vi "Dashboard Main.vi"() -> ()   [LabVIEW 2017]
uses:
  <vilib>/Utility/miscctls.llb/LVRowAndColumnTypeDef.ctl
  <vilib>/event_ctls.llb/eventvkey.ctl
  <vilib>/Rock Robotics/Network Tables/NT Read Numeric Array.vi
  <vilib>/Rock Robotics/WPI/Dashboard/WPI_DashboardLogging Global.vi
panel:
  in  "Camera Settings Right":T1={"Frame Rate"=30, "Compression"=30, "Size"=1, "DB Camera Config"=FALSE} {"Frame Rate" scale=1.0..30.0; "Compression" scale=100.0..-1.0; "Size" items=["640x480", "320x240", "160x120"]}
  in  "Camera Name Right":string(combo)="No Camera Selection"
  out "Camera Info":cluster{"Mbps LED":bool, "Mbps":dbl, "fps":dbl} {"fps" format="%#.1g"; "Mbps" format="%#.1g"}
  in  "Camera Settings":T1={"Frame Rate"=30, "Compression"=30, "Size"=1, "DB Camera Config"=FALSE} {"Frame Rate" scale=1.0..30.0; "Compression" scale=100.0..-1.0; "Size" items=["640x480", "320x240", "160x120"]}
  in  "TCP":refnum<k5>
  in  "Rec Mode":enum32{"Stop", "Record", "Playback"}(radio)
  out "Robot IP":string
  out "Image Message":string="Timeout in Camera Communications"
  in  "Dashboard Tab":T2(tab)
  out "Pitch":dbl
  out "Roll":dbl
  in  "Select Auto":string(combo)="Select Autonomous ..."
  out "NT Connection":bool
  out "MotorChart R":cluster{"Numeric":dbl, "Numeric":dbl}(graph)
  out "MotorChart L":cluster{"Numeric":dbl, "Numeric":dbl}(graph)
  out "MotorSliders R":cluster{"MotorSlide1":dbl, "MotorSlide2":dbl} {"MotorSlide2" scale=-1.0..1.0 scale format="%#_2e"; "MotorSlide1" scale=-1.0..1.0 scale format="%#_2e"}
  out "MotorSliders L":cluster{"MotorSlide1":dbl, "MotorSlide2":dbl} {"MotorSlide2" scale=-1.0..1.0 scale format="%#_2e"; "MotorSlide1" scale=-1.0..1.0 scale format="%#_2e"}
  out "Yaw":dbl
  out "JS1 Z":dbl(slide) scale=-1.0..1.0 scale format="%#_2e"
  out "JS1 Graph":cluster{"X":dbl, "Y":dbl}[](graph)
  out "JS1 Buttons":T3
  out "JS2 Z":dbl(slide) scale=-1.0..1.0 scale format="%#_2e"
  out "JS2 Graph":cluster{"X":dbl, "Y":dbl}[](graph)
  out "JS2 Buttons":T3
  out "Mode":T4(ring)=enum."Auto Disabled"
  out "Camera Image Right":T5(plugin-control)
  in  "DB/String 9":string
  in  "DB/String 8":string
  in  "DB/String 7":string
  in  "DB/String 6":string
  in  "DB/String 5":string
  in  "DB/String 4":string
  in  "DB/String 3":string
  in  "DB/String 2":string
  in  "DB/String 1":string
  in  "DB/String 0":string
  in  "DB/Slider 0":dbl(slide) scale=0.0..5.0
  in  "DB/Slider 1":dbl(slide) scale=0.0..5.0
  in  "DB/Slider 2":dbl(slide) scale=0.0..5.0
  in  "DB/Slider 3":dbl(slide) scale=0.0..5.0
  out "DB/LED 3":bool
  out "DB/LED 2":bool
  out "DB/LED 1":bool
  out "DB/LED 0":bool
  in  "DB/Button 3":bool
  in  "DB/Button 2":bool
  in  "DB/Button 1":bool
  in  "DB/Button 0":bool caption="New Name"
  in  "Test Slider":dbl(slide) scale=0.0..100.0 scale format="%#_3g"
  in  "On/Off":bool caption="Solenoid"
  in  "Test Name":u16(ring) items=["Select the test to run..."]
  in  "Test Tree":string(tree)
  in  "Motor":cluster{"Value":dbl, "Enable":bool} {"Value" scale=-1.0..1.0 scale format="%#_3g"}
  out "Progress":T6 {"Test Progress" scale=0.0..100.0}
  in  "Rev/Fwd":cluster{"Forward":bool, "Reverse":bool}
  in  "Test Ring":u16(ring) items=["Monochrome", "Color"]
  out "Cmd Status":string
  in  "Execute Command":bool
  in  "Command Params":string[][](table)
  in  "Command Selection":i32(listbox)
  in  "CheckList":i32(listbox)
  out "Tree":string(tree)
  out "Camera Image":T5(plugin-control)
  out "Background":bool
  in  "Camera Name":string(combo)="No Camera Selection"
  # "HW"
  # "HW"
  # "Joysticks"
  # "Drive Motors"
  # "Front"
  # "Right"
  # "Left"
  # "Back"
  # "This tab is a great place for autonomous settings and robot-specific values.\nPlace controls and indicators inside this tab and match name to\nDashboard Variables on robot. You can also delete this comment."
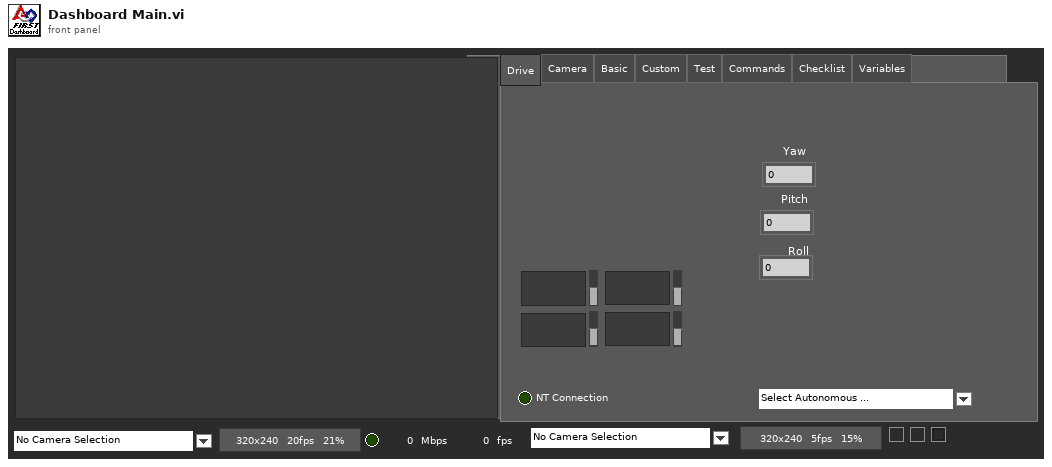
[diagram p1: front panel]
types:
  T1 = cluster{"Frame Rate":i32, "Compression":i32, "Size":u16, "DB Camera Config":bool}
  T2 = enum32{"Drive", "Camera", "Basic", "Custom", "Test", "Commands", "Checklist", "Variables"}
  T3 = cluster{bool, bool, bool, bool, bool, bool, bool, bool, bool, bool, bool, bool}
  T4 = enum8{"Tele-Op Disabled", "Tele-Op Enabled", "Auto Disabled", "Auto Enabled", "Test Disabled", "Test Enabled", "Disconnected", "No Code", "E-Stop"}
  T5 = typedef "IMAQ Image.ctl" = refnum<image>
  T6 = cluster{"Test Progress":u8, "Test Progress Text":string}
  T7 = cluster{"Save Path":path, "Interval (s)":dbl, "Keep":i32}
  T8 = typedef "Image Type" = u32
  T9 = cluster{"IDs":cluster{"RPC field ID":u16, "Unique ID":u16}, "String":string}
  T10 = cluster{"Camera Name":string, string, "Saved DB Images Info":cluster{"Save Path":path, "Interval (s)":dbl, "Keep":i32}}
  T11 = cluster{"Camera Name Right":string, string, "Saved DB Images Info":cluster{"Save Path":path, "Interval (s)":dbl, "Keep":i32}}
  T12 = cluster{"Camera Image":refnum<vi>, "Dashboard Tab":refnum<vi>, "Background":refnum<vi>, "Rec Mode":refnum<vi>, "Test Slider":refnum<vi>, "On/Off ":refnum<vi>, "Test Ring":refnum<vi>, "Rev/Fwd":refnum<vi>, "Test Name":refnum<vi>, "Motor":refnum<vi>, "Progress":refnum<vi>, "CheckList":refnum<vi>, "Tree":refnum<vi>, "Test Tree":refnum<vi>, "Command Params":refnum<vi>, "Command Selection":refnum<vi>, "Execute Command":refnum<vi>, "Cmd Status":refnum<vi>, "Camera Settings":refnum<vi>, "Camera Name":refnum<vi>, "Camera Info":refnum<vi>, "Camera Settings Right":refnum<vi>, "Camera Name Right":refnum<vi>, "Camera Image Right":refnum<vi>}
  T13 = cluster{"Error Strings":string, "Disable Counts":cluster{u16, u16}, "Rail Faults":cluster{u16, u16, u16}, "Robot IP":string, "DB Mode":u8, "Event Info":cluster{"Name":string, "Type":u8, "Number":u16, "Replay":u8}}
  T14 = cluster{"Storage":cluster{"Disk Free":u64, "RAM Block":u32, "RAM free":u32}, "CPU Utilization":cluster{"CPU % ISR":sgl, "CPU % Time Crit":sgl, "CPU % Timed Str":sgl, "CPU % High":sgl, "CPU % Above":sgl, "CPU % Normal":sgl, "CPU % Low":sgl}, "CAN":cluster{"% Bus Utilization":sgl, "Bus Off Cnt":u32, "TX_FIFO Full Cnt":u32, "Receive Error Cnt":u8, "Transmit Error Cnt":u8}, "HID":cluster{"HID Outputs":u32, "Rumble Low":u16, "Rumble High":u16}[]}
  T15 = cluster{"Status bits":cluster{"Test Mode":bool, "Autonomous":bool, "Enabled":bool, "Code Start":bool, "Brownout":bool, "Reserved 2":bool, "Reserved 3":bool, "E-Stop":bool}, "Code Trace":cluster{"Disabled":bool, "TeleOp":bool, "Auto":bool, "Test":bool}, "Controller Type":enum16{"unknown", "cRIO", "roboRio"}, "Code?":enum16{"unknown", "noCode", "code"}, "Battery V":dbl}
  T16 = cluster{"Control Bits":cluster{"TestMode":bool, "Autonomous":bool, "Enabled":bool, "FMS Present":bool, bool, bool, bool, "E-Stop":bool}, "Team Station ":u8, "Countdown":sgl, "Joystick Values":cluster{"Axes":dbl[], "Buttons":bool[], "POVs":i16[]}[]}
  T17 = cluster{"Axes":dbl[], "Buttons":bool[], "POVs":i16[]}[]
  T18 = cluster{"Axes":dbl[], "Buttons":bool[], "POVs":i16[]}
  T19 = cluster{"Buttons[0]":bool, "Buttons[1]":bool, "Buttons[2]":bool, "Buttons[3]":bool, "Buttons[4]":bool, "Buttons[5]":bool, "Buttons[6]":bool, "Buttons[7]":bool, "Buttons[8]":bool, "Buttons[9]":bool, "Buttons[10]":bool, "Buttons[11]":bool}
  T20 = cluster{"Operation":enum16{"Update", "Clear"}, "Color Box":u32}[]
  T21 = typedef "eventvkey.ctl" = enum16{"ASCII", "Enter", "Return", "Shift", "Ctrl", "Alt", "Cmd", "Opt", "Caps", "NumLock", "Clear", "Break", "Up", "Down", "Left", "Right", "Insert", "Delete", "Home", "End", "PageUp", "PageDown", "Escape", "Help", "Pause", "ScrollLock", "F1", "F2", "F3", "F4", "F5", "F6", "F7", "F8", "F9", "F10", "F11", "F12", "F13", "F14", "F15", "F16", "F17", "F18", "F19", "F20", "F21", "F22", "F23", "F24", "Play", "VolumeUp", "VolumeDown", "Mute", "Two Byte Char"}
  T22 = cluster{"Image Size":bool, "Image Type":bool, "Pixel Value":bool, "ROI Information":bool, "Zoom Factor":bool}
  T23 = cluster{"Operation":enum16{"Update", "Clear"}, "Color Box":u32}
  T24 = typedef "LVRowAndColumnTypeDef.ctl" = cluster{"Row":i32, "Column":i32}
  T25 = cluster{"Shift":bool, "Ctrl":bool, "Alt":bool, "Cmd":bool, "Opt":bool}
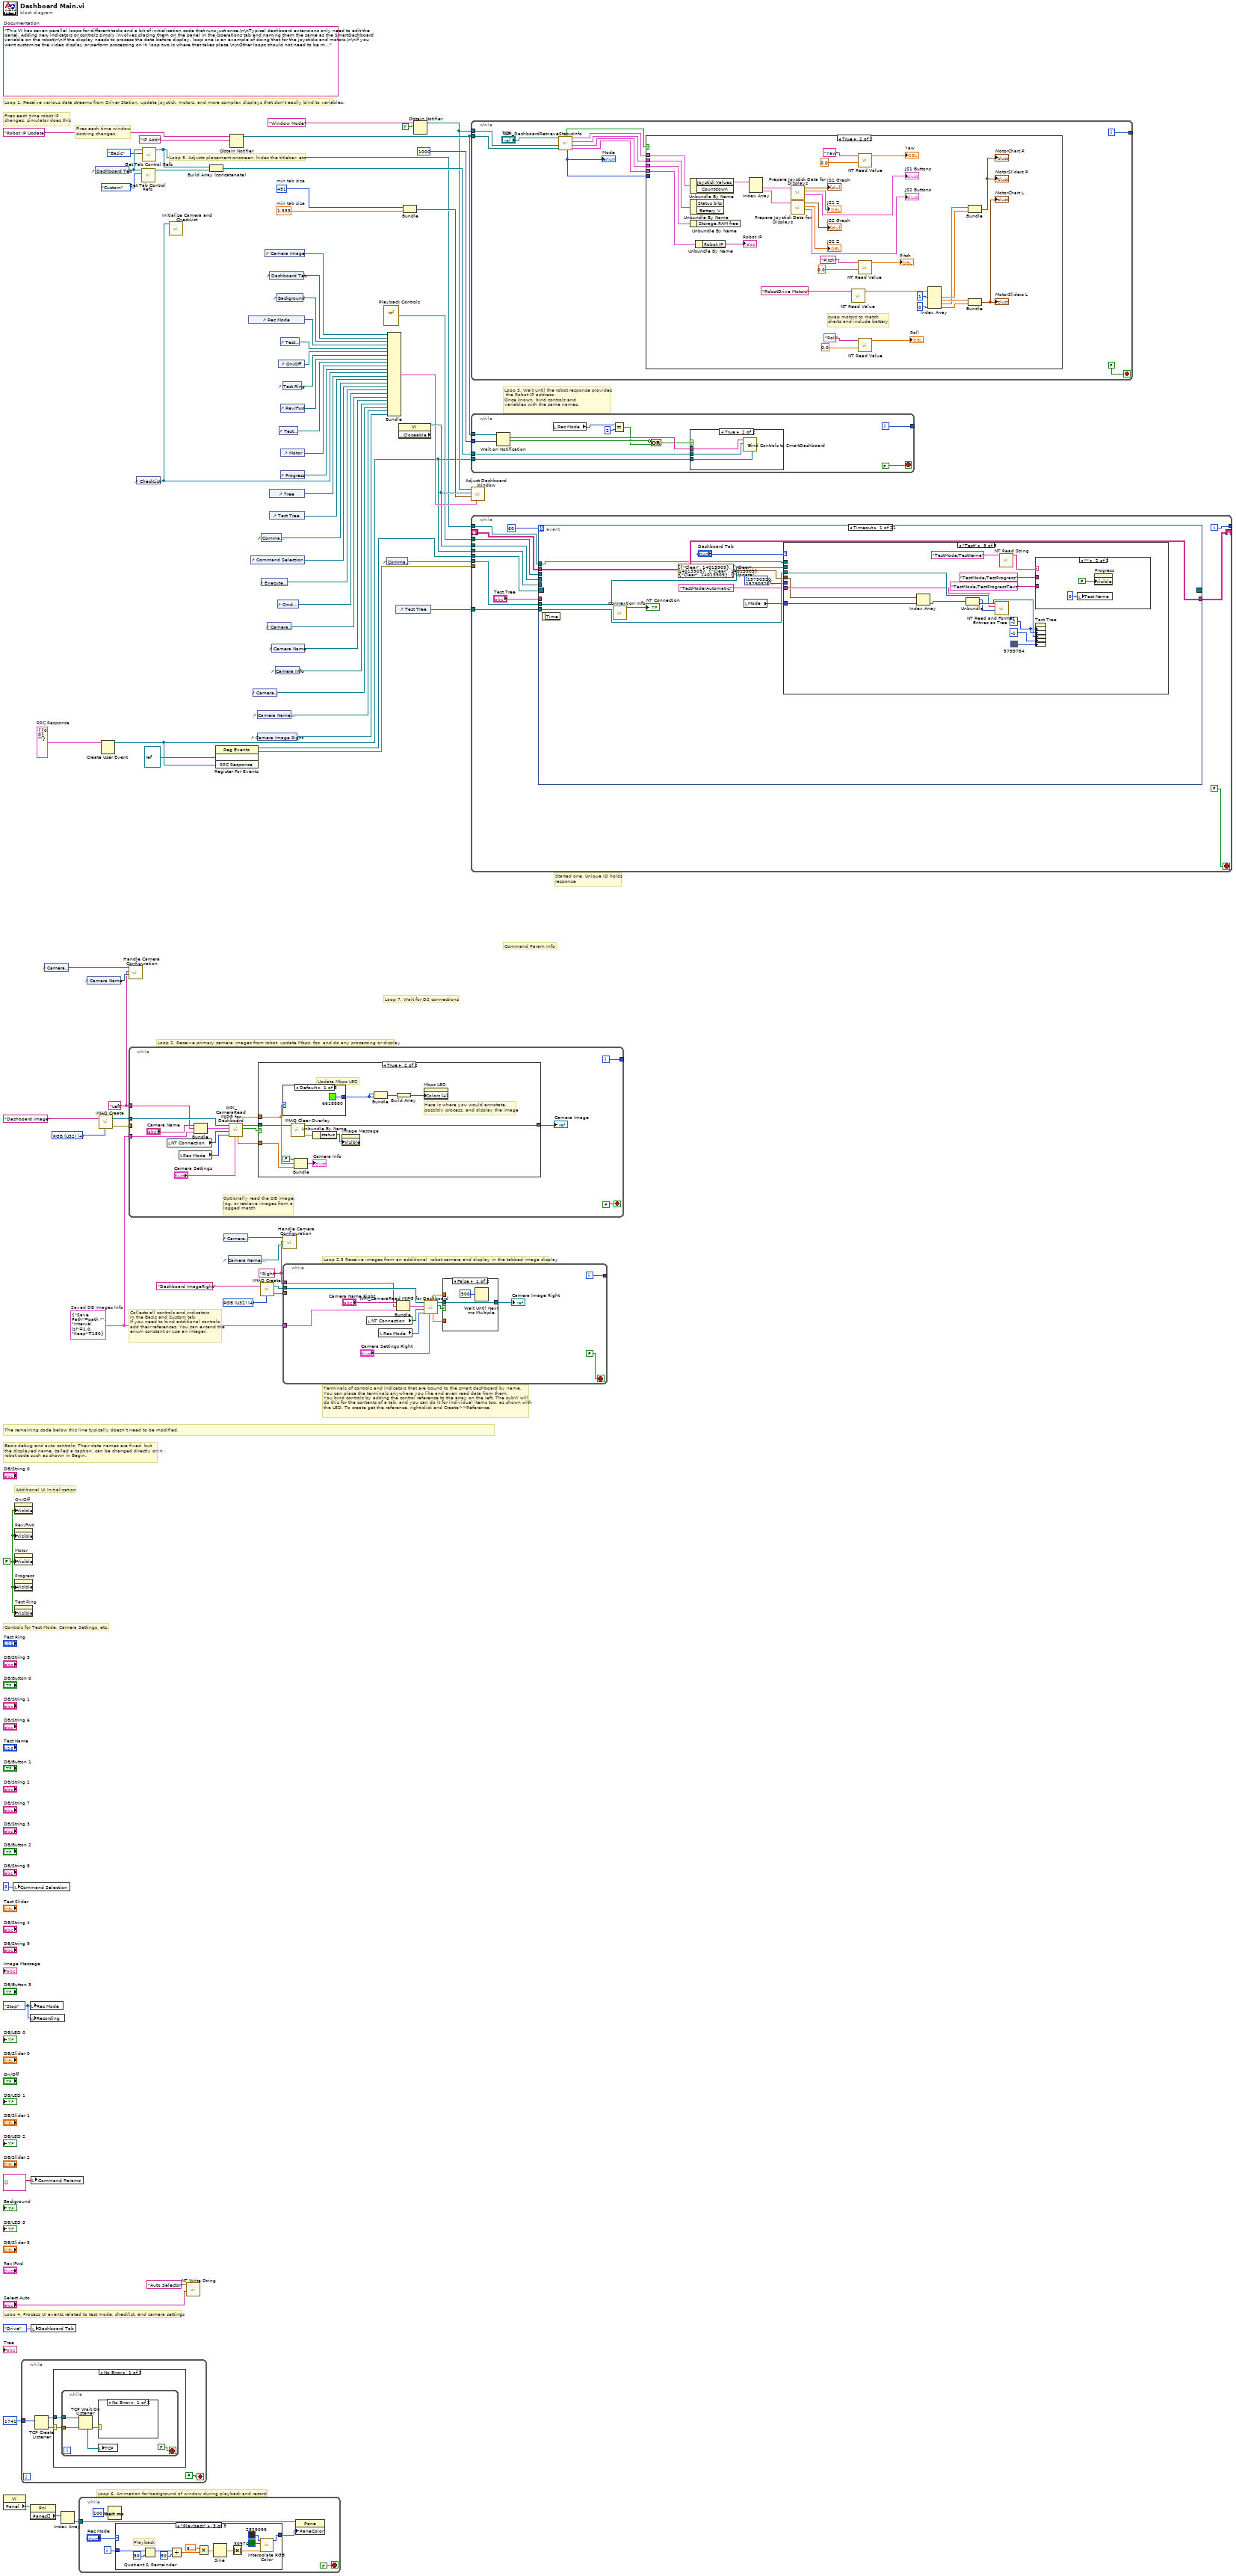
[diagram p0: block diagram]
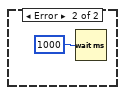
[diagram p3: hidden frame]
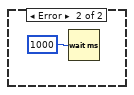
[diagram p4: hidden frame]
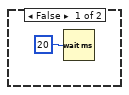
[diagram p5: hidden frame]
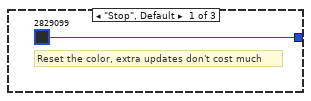
[diagram p6: hidden frame]
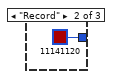
[diagram p7: hidden frame]
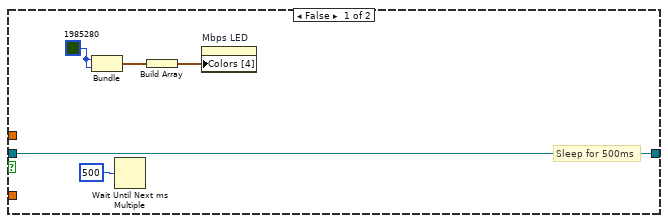
[diagram p9: hidden frame]
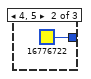
[diagram p10: hidden frame]
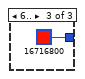
[diagram p11: hidden frame]
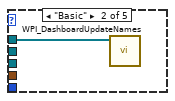
[diagram p13: hidden frame]
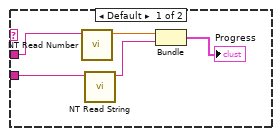
[diagram p14: hidden frame]
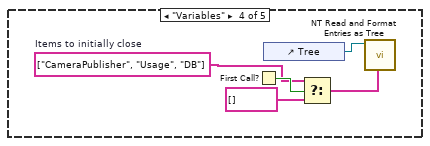
[diagram p15: hidden frame]
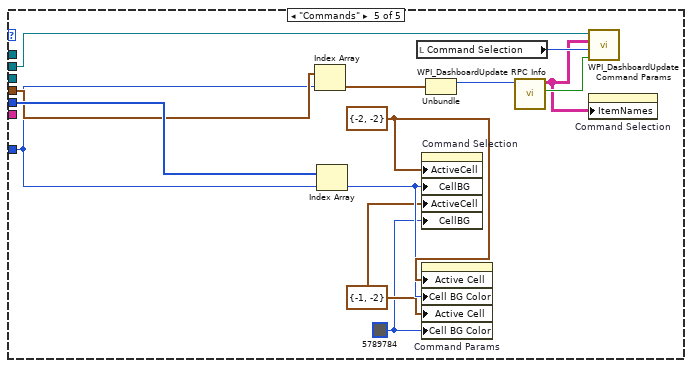
[diagram p16: hidden frame]
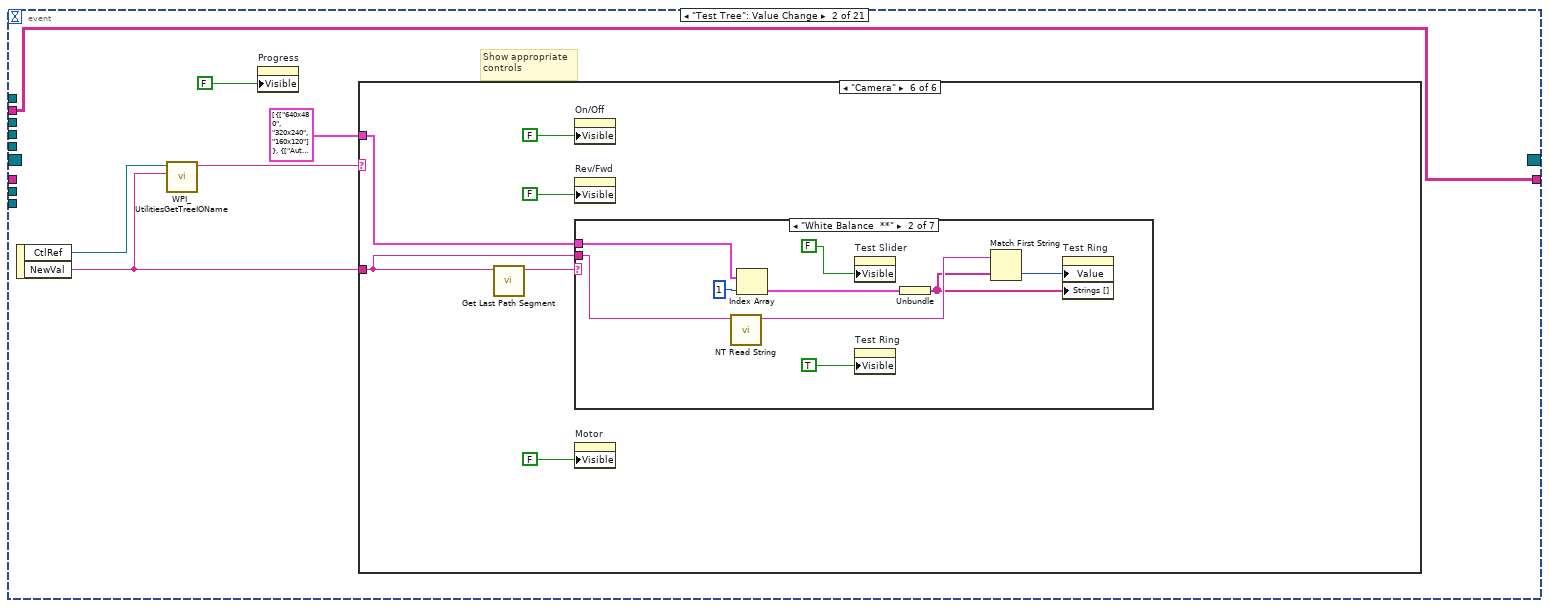
[diagram p17: hidden frame]
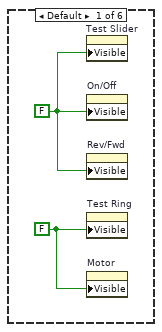
[diagram p18: hidden frame]
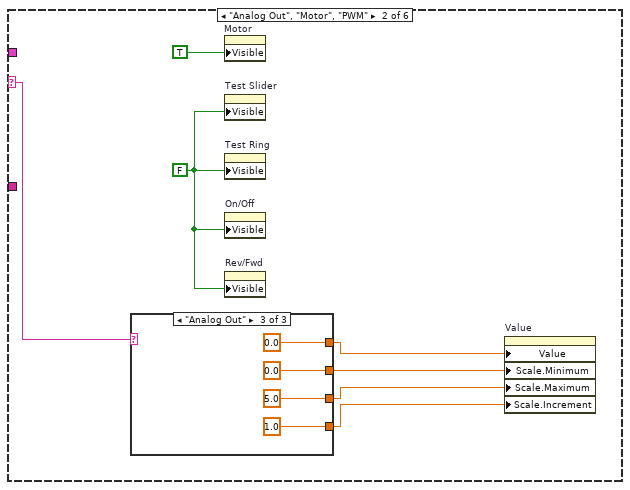
[diagram p19: hidden frame]
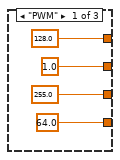
[diagram p20: hidden frame]
diagram:
  w3 = T7 {"Save Path"=path "", "Interval (s)"=1.0, "Keep"=180}  # Saved DB Images Info
  w2 = "Right"
  w1 = "Left"
  w13 = T8 4 items=["Grayscale (U8)", "Grayscale (I16)", "Grayscale (SGL)", "Complex (CSG)", "RGB (U32)", "HSL (U32)", "RGB (U64)"] ("Image Type")
  w29 = T9 {"IDs"={"RPC field ID"=0, "Unique ID"=0}, "String"=""}  # RPC Response
  w52 = 491  # min tab size
  w51 = 1.333  # min tab size
  w59 = enum32{"Stop", "Record", "Playback"}."Stop" ("Rec Mode")
  w36 = FALSE ("Visible")
  (unwired) "This VI has seven parallel loops for different tasks and a bit of initialization code that runs just once.\n\nTypical dashboard extensions only need to edit the panel. Adding new indicators or controls simply involves placing them on the panel in the Operations tab and naming them the same as the SmartDashboard variable on the robot\n\nIf the display needs to process the data before display, loop one is an example of doing that for the joysticks and motors.\n\nIf you want customize the video display or perform processing on it, loop two is where that takes place.\n\nOther loops should not need to be modified. They are pretty standard, and document the task they perform."  # Documentation
  w76 = T8 4 items=["Grayscale (U8)", "Grayscale (I16)", "Grayscale (SGL)", "Complex (CSG)", "RGB (U32)", "HSL (U32)", "RGB (U64)"] ("Image Type")
  # "Loop 2.5 Receive images from an additional  robot camera and display in the tabbed image display"
  # "Command Param Info"
  # "Started one, Unique ID holds\nresponse"
  # "Loop 7. Wait for DS connections"
  # "Basic debug and auto controls: Their data names are fixed, but\nthe displayed name, called a caption, can be changed directly or in\nrobot code such as shown in Begin."
  # "Controls for Test Mode, Camera Settings, etc."
  # "Additional UI Initialization"
  # "Loop 6. Animation for background of window during playback and record"
  # "Fires each time robot IP\nchanges, simulator does this"
  # "Fires each time window\ndocking changes."
  # "Collects all controls and indicators\nin the Basic and Custom tab.\nIf you need to bind additional controls,\nadd their references. You can extend the\nenum constant or use an integer."
  # "The remaining code below this line typically doesn't need to be modified."
  # "Loop 4. Process UI events related to test mode, checklist, and camera settings"
  # "Terminals of controls and indicators that are bound to the smart dashboard by name.\nYou can place the terminals anywhere you like and even read data from them.\nYou bind controls by adding the control reference to the array on the left. The subVI will\ndo this for the contents of a tab, and you can do it for individual items too, as shown with\nthe LED. To create get the reference, right-click and Create>>Reference."
  # "Loop 3. Wait until the robot response provides\n the Robot IP address.\nOnce known, bind controls and\nvariables with the same names."
  # "Loop 5. Adjusts placement onscreen, hides the titlebar, etc."
  # "Loop 1. Receive various data streams from Driver Station, update joystick, motors, and more complex displays that don't easily bind to variables."
  # "Loop 2. Receive primary camera images from robot, update Mbps, fps, and do any processing or display"
  n1 = property class="VI"() -> ("Panel"=w66:refnum<vi>)  [unwired: 2 in, 2 out]
  n2 = local write "Command Selection"(u16 0 ("milliseconds to wait")) -> ()
  n3 = property on="On/Off" class="Bool (strict)"("Visible"=w36) -> ()  [unwired: 2 in, 2 out]
  n4 = property on="Rev/Fwd" class="Clust (strict)"("Visible"=w36) -> ()  [unwired: 2 in, 2 out]
  n5 = property on="Motor" class="Clust (strict)"("Visible"=w36) -> ()  [unwired: 2 in, 2 out]
  n6 = property on="Progress" class="Clust (strict)"("Visible"=w36) -> ()  [unwired: 2 in, 2 out]
  n7 = property on="Test Ring" class="Ring (strict)"("Visible"=w36) -> ()  [unwired: 2 in, 2 out]
  n8 = while {
    tunnel: u16 1741 ("timeout ms (25000)") -> [w78]
    stop <- FALSE stop-if-true
    n9 = TCP Create Listener(10:w78) -> (0:w77:errorcluster, 3:w79:refnum<k5>)  [unwired: 4 in, 1 out]
    n10 = case shown="No Error" w77 {
      selector: w77 -> [w81 _]
      tunnel: w79 -> [w82 _]
      frame No Error {
        n11 = while {
          tunnel: w82 -> [w85]
          tunnel: w81 -> [w84]
          stop <- FALSE stop-if-true
          n12 = TCP Wait On Listener(8:w84, 11:w85) -> (0:w86:errorcluster, 4:w87:refnum<k5>)  [unwired: 2 in, 3 out]
          n13 = case shown="No Error" w86 {
            frame No Error {
            }
            frame Error {
              n14 = Wait (ms)(milliseconds to wait=u32 1000) -> ()  [unwired: 1 out]
            }
          }
          n15 = local write "TCP"(w87) -> ()
        }
      }
      frame Error {
        n16 = Wait (ms)(milliseconds to wait=u32 1000) -> ()  [unwired: 1 out]
      }
    }
  }
  n17 = local write "Rec Mode"(w59) -> ()
  n18 = global write "WPI_DashboardLogging Global.vi" "Recording"(w59) -> ()
  n19 = property class="Pnl"(reference=w66) -> ("Panes[]"=w67:refnum<vi>[])  [unwired: 1 in, 2 out]
  n20 = local write "Command Params"(string[][] [] ("Command Params")) -> ()
  n21 = local write "Dashboard Tab"(T2."Drive" ("Dashboard Tab")) -> ()
  n22 = control-ref of="Camera Settings"() -> (w22:refnum<vi>)
  n23 = Index Array(array=w67) -> (element=w65:refnum<vi>)  [unwired: 1 in]
  n24 = while {
    tunnel: w65 -> [w91]
    i -> [w94]
    stop <- FALSE stop-if-true
    n25 = Wait (ms)(milliseconds to wait=u32 100) -> ()  [unwired: 1 out]
    n26 = case shown="\"Playback\"" "Rec Mode" {
      tunnel: w94 -> [_ _ w109]
      tunnel: [u32 2829099 ("Base Color") u32 11141120 ("Target Color") w98] -> w90
      frame "Stop", Default {
        # "Reset the color, extra updates don't cost much"
      }
      frame "Record" {
      }
      frame "Playback" {
        # "Playback"
        n27 = Quotient & Remainder(x=w109, y=u32 50 ("milliseconds to wait")) -> (x-y*floor(x/y)=w105:u32)  [unwired: 1 out]
        n28 = Divide(x=w105, y=u32 50 ("milliseconds to wait")) -> (x/y=w102:dbl)
        n29 = Multiply(x=6.283185307179586, y=w102) -> (x*y=w107:dbl)
        n30 = Sine(x=w107) -> (sin(x)=w106:dbl)
        n31 = Absolute Value(x=w106) -> (abs(x)=w99:dbl)
        n32 = call "Interpolate RGB Color.vi"("Proportion"=w99, "Target Color"=u32 30976, "Base Color"=u32 2829099) -> ("Result Color"=w98:u32)  [unwired: 8 in]
      }
    }
    n33 = property class="Pane"(reference=w91, "PaneColor"=w90) -> ()  [unwired: 1 in, 2 out]
  }
  n34 = control-ref of="Camera Name"() -> (w21:refnum<vi>)
  n35 = control-ref of="Dashboard Tab"() -> (w57:refnum<vi>)
  n36 = call "IMAQ Create"("Image Name"="Dashboard Image", "Image Type"=w76) -> ("New Image"=w74:T5, "error out"=w73:errorcluster)  [unwired: 2 in, 1 out]
  n37 = Create User Event(user event datatype=w29) -> (user event=w25:refnum<user-event>)  [unwired: 1 in, 1 out]
  n38 = call "Handle Camera Configuration.vi"("CameraNameRef"=w21, "Display Name"=w1, "ClusterRef"=w22) -> ()  [unwired: 9 in]
  n39 = while {
    tunnel: w74 -> [w122]
    tunnel: w73 -> [_]
    tunnel: [w123] -> _
    tunnel: w3 -> [w113]
    tunnel: w1 -> [w110]
    i -> [w123]
    stop <- FALSE stop-if-true
    # "Optionally read the DB image,\nlog, or retrieve images from a\nlogged match"
    n40 = local read "NT Connection"() -> (w114:bool)
    n41 = local read "Rec Mode"() -> (w118:enum32{"Stop", "Record", "Playback"})
    n42 = Bundle("Camera Name"="Camera Name", w110, "Saved DB Images Info"=w113) -> (w112:T10)  [unwired: 1 in]
    n43 = call <vilib>:"WPI_CameraRead MJPG for Dashboard.vi"("Camera Settings"="Camera Settings", "Rec Mode"=w118, "NT Connection"=w114, "Capture Info"=w112, "Refnum in"=w122) -> ("Active"=w120:bool, "Refnum out"=w121:T5, "FPS"=w119:dbl, "Bandwidth (Mbps)"=w117:dbl)  [unwired: 3 in]
    n44 = case shown="True" w120 {
      tunnel: w121 -> [w125 w136]
      tunnel: w117 -> [_ w133]
      tunnel: w119 -> [_ w134]
      tunnel: [w125 w130] -> w115
      frame False {
        w127 = u32 1985280 ("Color Box")
        # "Sleep for 500ms"
        n45 = Bundle("Color Box"=w127, "Color Box"=w127) -> (w128:cluster{"Color Box":u32, "Color Box":u32})  [unwired: 1 out]
        n46 = Wait Until Next ms Multiple(millisecond multiple=u32 500) -> ()  [unwired: 1 out]
        n47 = Build Array(w128) -> (w126:cluster{"Color Box":u32, "Color Box":u32}[])
        n48 = property on="Mbps LED" class="Bool (strict)"("Colors [4]"=w126) -> ()  [unwired: 2 in, 2 out]
      }
      frame True {
        # "Here is where you would annotate,\npossibly process, and display the image"
        # "Update Mbps LED"
        n49 = case shown="Default" w133 {
          tunnel: [u32 6618880 ("Color Box") u32 16776722 ("Color Box") u32 16716800 ("Color Box")] -> w137
          frame Default {
          }
          frame 4, 5 {
          }
          frame 6.. {
          }
        }
        n50 = call "IMAQ Clear Overlay"("Image"=w136) -> ("error out"=w139:errorcluster, "Image Out"=w130:T5)  [unwired: 2 in, 7 out]
        n51 = Bundle(FALSE, "Bandwidth (Mbps)"=w133, "FPS"=w134) -> (→"Camera Info":cluster{bool, "Bandwidth (Mbps)":dbl, "FPS":dbl})  [unwired: 1 in]
        n52 = Unbundle By Name(w139) -> ("status"=w140:bool)
        n53 = property on="Image Message" class="Str"("Visible"=w140) -> ()  [unwired: 2 in, 2 out]
        n54 = Bundle("Color Box"=w137, "Color Box"=w137) -> (w138:cluster{"Color Box":u32, "Color Box":u32})  [unwired: 1 out]
        n55 = Build Array(w138) -> (w135:cluster{"Color Box":u32, "Color Box":u32}[])
        n56 = property on="Mbps LED" class="Bool (strict)"("Colors [4]"=w135) -> ()  [unwired: 2 in, 2 out]
      }
    }
    "Camera Image" <- w115
  }
  n57 = control-ref of="CheckList"() -> (w47:refnum<vi>)
  n58 = call <vilib>:"Get Tab Control Refs.vi"("Page Index"=T2."Custom" ("Dashboard Tab"), "TabControl in"=w57) -> ("ControlsOnPage"=w56:refnum<vi>[])  [unwired: 9 in]
  n59 = call <vilib>:"Get Tab Control Refs.vi"("Page Index"=T2."Basic" ("Dashboard Tab"), "TabControl in"=w57) -> ("ControlsOnPage"=w17:refnum<vi>[])  [unwired: 9 in]
  n60 = call "Initialize Camera and CheckList.vi"("ListBox in"=w47) -> ()  [unwired: 11 in]
  n61 = call <vilib>:"NT Write String.vi"("String"="Select Auto", "Name"="Auto Selector") -> ()  [unwired: 9 in, 1 out]
  n62 = Build Array (concatenate)(w17, w56) -> (w55:refnum<vi>[])
  n63 = register-events(refnum<vi> refnum, w25) -> (reference out=w63:refnum<event-registration>, error out=w62:errorcluster)  [unwired: 2 in]
  n64 = control-ref of="Camera Settings Right"() -> (w10:refnum<vi>)
  n65 = control-ref of="Camera Name Right"() -> (w9:refnum<vi>)
  n66 = Obtain Notifier(name (unnamed)="Robot IP Update", notification data type="IP Addr" ("name (unnamed)")) -> (notifier out=w35:refnum<notifier>)  [unwired: 2 in, 2 out]
  n67 = control-ref of="Rec Mode"() -> (w42:refnum<vi>)
  n68 = control-ref of="Command Selection"() -> (w28:refnum<vi>)
  n69 = control-ref of="Camera Settings Right"() -> (w8:refnum<vi>)
  n70 = control-ref of="Camera Name Right"() -> (w7:refnum<vi>)
  n71 = control-ref of="Camera Image Right"() -> (w6:refnum<vi>)
  n72 = call "IMAQ Create"("Image Name"="Dashboard ImageRight", "Image Type"=w13) -> ("New Image"=w12:T5, "error out"=w11:errorcluster)  [unwired: 2 in, 1 out]
  n73 = control-ref of="Command Params"() -> (w31:refnum<vi>)
  n74 = control-ref of="Execute Command"() -> (w30:refnum<vi>)
  n75 = control-ref of="Camera Image"() -> (w54:refnum<vi>)
  n76 = control-ref of="Camera Settings"() -> (w20:refnum<vi>)
  n77 = control-ref of="Dashboard Tab"() -> (w53:refnum<vi>)
  n78 = control-ref of="Tree"() -> (w46:refnum<vi>)
  n79 = control-ref of="Test Tree"() -> (w45:refnum<vi>)
  n80 = control-ref of="Camera Name"() -> (w19:refnum<vi>)
  n81 = control-ref of="Camera Info"() -> (w18:refnum<vi>)
  n82 = control-ref of="Background"() -> (w49:refnum<vi>)
  n83 = control-ref of="Cmd Status"() -> (w24:refnum<vi>)
  n84 = control-ref of="On/Off"() -> (w40:refnum<vi>)
  n85 = control-ref of="Test Name"() -> (w44:refnum<vi>)
  n86 = control-ref of="Test Slider"() -> (w41:refnum<vi>)
  n87 = control-ref of="Rev/Fwd"() -> (w38:refnum<vi>)
  n88 = control-ref of="Motor"() -> (w43:refnum<vi>)
  n89 = control-ref of="Progress"() -> (w37:refnum<vi>)
  n90 = control-ref of="Test Ring"() -> (w39:refnum<vi>)
  n91 = call "Handle Camera Configuration.vi"("CameraNameRef"=w9, "Display Name"=w2, "ClusterRef"=w10) -> ()  [unwired: 9 in]
  n92 = while {
    tunnel: w12 -> [w158]
    tunnel: w11 -> [_]
    tunnel: [w153] -> _
    tunnel: w3 -> [w147]
    tunnel: w2 -> [w144]
    i -> [w153]
    stop <- FALSE stop-if-true
    n93 = local read "NT Connection"() -> (w148:bool)
    n94 = local read "Rec Mode"() -> (w157:enum32{"Stop", "Record", "Playback"})
    n95 = Bundle("Camera Name Right"="Camera Name Right", w144, "Saved DB Images Info"=w147) -> (w146:T11)  [unwired: 1 in]
    n96 = call <vilib>:"WPI_CameraRead MJPG for Dashboard.vi"("Camera Settings"="Camera Settings Right", "Rec Mode"=w157, "NT Connection"=w148, "Capture Info"=w146, "Refnum in"=w158) -> ("Active"=w152:bool, "Refnum out"=w155:T5, "FPS"=w150:dbl, "Bandwidth (Mbps)"=w151:dbl)  [unwired: 3 in]
    n97 = case shown="False" w152 {
      tunnel: w155 -> [w159 w161]
      tunnel: w151 -> [_ _]
      tunnel: w150 -> [_ _]
      tunnel: [w159 w161] -> w149
      frame False {
        n98 = Wait Until Next ms Multiple(millisecond multiple=u32 500) -> ()  [unwired: 1 out]
      }
      frame True {
      }
    }
    "Camera Image Right" <- w149
  }
  n99 = vi-ref "Playback Controls.vi"() -> (w64:refnum<vi>)
  n100 = control-ref of="Command Params"() -> (w23:refnum<vi>)
  n101 = Bundle("Camera Image"=w54, "Dashboard Tab"=w53, "Background"=w49, "Rec Mode"=w42, "Test Slider"=w41, "On/Off"=w40, "Test Ring"=w39, "Rev/Fwd"=w38, "Test Name"=w44, "Motor"=w43, "Progress"=w37, "CheckList"=w47, "Tree"=w46, "Test Tree"=w45, "Command Params"=w31, "Command Selection"=w28, "Execute Command"=w30, "Cmd Status"=w24, "Camera Settings"=w20, "Camera Name"=w19, "Camera Info"=w18, "Camera Settings Right"=w8, "Camera Name Right"=w7, "Camera Image Right"=w6) -> (w48:T12)  [unwired: 1 in]
  n102 = control-ref of="Test Tree"() -> (w68:refnum<vi>)
  n103 = property class="VI" props=["Front Panel.Closeable"]() -> (reference out=w58:refnum<vi>)  [unwired: 2 in, 2 out]
  n104 = Bundle("min tab size"=w52, "min tab size"=w51) -> (w50:cluster{"min tab size":i32, "min tab size":dbl})  [unwired: 1 in]
  n105 = Obtain Notifier(name (unnamed)="Window Mode", notification data type=TRUE) -> (notifier out=w34:refnum<notifier>)  [unwired: 2 in, 2 out]
  n106 = while {
    tunnel: [w171] -> _
    tunnel: w35 -> [w165]
    tunnel: w34 -> [w162]
    i -> [w171]
    stop <- FALSE stop-if-true
    n107 = call <vilib>:"WPI_DashboardRetrieveStatusInfo.vi"("Binding Refnum"=w165, "Window Mode Notifier"=w162, "TCP Cnx"="TCP") -> ("Power and Errors"=w166:T13, "Robot Metrics"=w169:T14, "Status Info"=w170:T15, "Control Info"=w167:T16, "Robot Mode"=w164:T4, "Process?"=w168:bool)  [unwired: 3 in]
    "Mode" <- w164
    n108 = case shown="True" w168 {
      tunnel: w170 -> [_ w206]
      tunnel: w169 -> [_ w205]
      tunnel: w167 -> [_ w204]
      tunnel: w166 -> [_ w203]
      tunnel: w164 -> [_ _]
      frame False {
        n109 = Wait (ms)(milliseconds to wait=u32 20) -> ()  [unwired: 1 out]
      }
      frame True {
        # "swap motors to match\ncharts and include battery"
        n110 = Unbundle By Name(w204) -> ("Joystick Values"=w194:T17)  [unwired: 1 out]
        n111 = Unbundle By Name(w206) -> ()  [unwired: 2 out]
        n112 = Unbundle By Name(w205) -> ()  [unwired: 1 out]
        n113 = Unbundle By Name(w203) -> ("Robot IP"=→"Robot IP":string)
        n114 = Index Array(array=w194) -> (element #1=w193:T18, element #2=w189:T18)  [unwired: 2 in]
        n115 = call "Prepare Joystick Data for Displays.vi"("Joystick Values"=w193) -> ("Buttons"=→"JS1 Buttons":T19, "Z Axis"=→"JS1 Z":dbl, "Cartesian Data"=→"JS1 Graph":cluster{"X axis":dbl, "X axis":dbl}[])  [unwired: 8 in]
        n116 = call "Prepare Joystick Data for Displays.vi"("Joystick Values"=w189) -> ("Buttons"=→"JS2 Buttons":T19, "Z Axis"=→"JS2 Z":dbl, "Cartesian Data"=→"JS2 Graph":cluster{"X axis":dbl, "X axis":dbl}[])  [unwired: 8 in]
        n117 = call-poly <vilib>:"NT Read Value.vi"("Name"="RobotDrive Motors") -> ("Numeric Array"=w184:dbl[])  [unwired: 9 in, 1 out]
        n118 = call-poly <vilib>:"NT Read Value.vi"("Default Value"=0.0, "Name"="Pitch") -> ("Numeric"=→"Pitch":dbl)  [unwired: 8 in, 1 out]
        n119 = call-poly <vilib>:"NT Read Value.vi"("Default Value"=0.0, "Name"="Yaw") -> ("Numeric"=→"Yaw":dbl)  [unwired: 8 in, 1 out]
        n120 = call-poly <vilib>:"NT Read Value.vi"("Default Value"=0.0, "Name"="Roll") -> ("Numeric"=→"Roll":dbl)  [unwired: 8 in, 1 out]
        n121 = Index Array(array=w184, index #1=1, index #4=0) -> (element #1=w198:dbl, element #2=w199:dbl, element #3=w197:dbl, element #4=w202:dbl)  [unwired: 2 in]
        n122 = Bundle("Numeric"=w197, "Numeric"=w198) -> (→"MotorChart R" →"MotorSliders R":cluster{"Numeric":dbl, "Numeric":dbl})  [unwired: 1 in]
        n123 = Bundle("Numeric"=w199, "Numeric"=w202) -> (→"MotorChart L" →"MotorSliders L":cluster{"Numeric":dbl, "Numeric":dbl})  [unwired: 1 in]
      }
    }
  }
  n124 = while {
    tunnel: w55 -> [w218]
    tunnel: w35 -> [w216]
    tunnel: [w214] -> _
    tunnel: u32 1000 ("milliseconds to wait") -> [w213]
    tunnel: w25 -> [w207]
    i -> [w214]
    stop <- FALSE stop-if-true
    n125 = Wait on Notification(notifier=w216, timeout in ms (-1)=w213) -> (notification=w215:string, timed out?=w211:bool)  [unwired: 2 in, 2 out]
    n126 = local read "Rec Mode"() -> (w209:enum32{"Stop", "Record", "Playback"})
    n127 = Equal?(x=w209, y=u16 2 ("Rec Mode")) -> (x = y?=w210:bool)
    n128 = Compound Arithmetic op=OR(invert w211, w210) -> (w212:bool)
    n129 = case shown="True" w212 {
      tunnel: w218 -> [_ w221]
      tunnel: w215 -> [_ w220]
      tunnel: w207 -> [_ w219]
      frame False {
      }
      frame True {
        n130 = call <vilib>:"Bind Controls to SmartDashboard.vi"("RPC ref"=w219, "Bound Control Refs"=w221, "Server IP Address"=w220) -> ()  [unwired: 9 in]
      }
    }
  }
  n131 = call "Adjust Dashboard Window.vi"("Sizing Refnums"=w48, "Size Constraints"=w50, "VI"=w58, "WIn Mode"=w34) -> ()  [unwired: 8 in]
  n132 = while {
    tunnel: [w231] -> _
    tunnel: w68 -> [w230]
    tunnel: w64 -> [w229]
    tunnel: w63 -> [w228]
    tunnel: w62 -> [_]
    tunnel: w58 -> [w227]
    tunnel: w25 -> [w226]
    tunnel: w23 -> [w225]
    shift-right: [w224] -> _
    shift-left: _ -> [w223]
    tunnel: w17 -> [w222]
    i -> [w231]
    stop <- FALSE stop-if-true
    n133 = event shown="[0] Timeout" {
      selector: w228 -> [_ _ _ _ _ _ _ _ _ _ _ _ _ _ _ _ _ _ _ _ _]
      dyn-events: [_ _ _ _ _ _ _ _ _ _ _ _ _ _ _ _ w491 _ _ _ _] -> _
      timeout: u32 60 ("milliseconds to wait") -> [_ _ _ _ _ _ _ _ _ _ _ _ _ _ _ _ _ _ _ _ _]
      tunnel: w230 -> [w243 _ _ _ _ _ _ _ _ _ _ _ _ _ _ _ _ _ _ _ _]
      tunnel: "Test Tree" -> [_ _ _ _ _ _ _ _ _ _ _ w458 w466 w468 w472 w480 _ _ _ _ _]
      tunnel: w229 -> [_ _ _ _ _ _ _ _ _ _ _ _ _ _ _ _ w493 _ w511 _ _]
      tunnel: w227 -> [_ _ _ _ _ _ _ _ _ _ _ _ _ _ _ _ w489 _ _ _ _]
      tunnel: w226 -> [_ _ _ _ _ _ _ _ _ _ _ _ _ _ _ _ w487 _ _ _ _]
      tunnel: w225 -> [w238 _ _ _ _ _ w409 _ _ _ _ _ _ _ _ _ _ _ _ _ _]
      tunnel: [w237 w286 w388 w393 w402 w406 w407 w416 w426 w433 w445 w457 w464 w467 w471 w479 w486 w506 w508 w512 w525] -> w224
      tunnel: w223 -> [w237 w286 w388 w393 w402 w406 w407 _ _ w433 w445 w457 w464 w467 w471 w479 w486 w506 w508 w512 w525]
      tunnel: w222 -> [w235 _ _ _ _ _ _ _ _ _ _ _ _ _ _ _ _ _ _ _ _]
      event Timeout {
        n134 = event-data() -> ()  [unwired: 1 in, 1 out]
        n135 = call <vilib>:"Connextion Info.vi"() -> ("Connected"=→"NT Connection":bool)  [unwired: 10 in, 1 out]
        n136 = local read "Mode"() -> (w240:T4)
        n137 = case shown="\"Test\"" "Dashboard Tab" {
          tunnel: w243 -> [_ _ w259 _ _]
          tunnel: "TestMode/Automatic/" ("Name Pattern") -> [_ _ w258 _ _]
          tunnel: T20 [{"Operation"=enum."Clear", "Color Box"=14013909}, {"Operation"=enum."Clear", "Color Box"=14013909}, {"Operation"=enum."Clear", "Color Box"=14013909}, {"Operation"=enum."Clear", "Color Box"=14013909}, {"Operation"=enum."Update", "Color Box"=14013909}, {"Operation"=enum."Update", "Color Box"=16777215}, {"Operation"=enum."Clear", "Color Box"=14013909}, {"Operation"=enum."Clear", "Color Box"=14013909}, {"Operation"=enum."Clear", "Color Box"=14013909}] -> [_ _ w251 _ w279]
          tunnel: w240 -> [_ _ w250 _ w278]
          tunnel: u32[] [15790320, 15790320, 15790320, 15790320, 16777215, 16777215, 15790320, 15790320, 15790320] -> [_ _ _ _ w284]
          tunnel: w238 -> [_ _ _ _ w272]
          tunnel: w235 -> [_ w245 _ _ _]
          frame "Custom", Default {
          }
          frame "Basic" {
            n138 = call <vilib>:"WPI_DashboardUpdateNames.vi"("Controls on Tab"=w245) -> ()  [unwired: 11 in]
          }
          frame "Test" {
            w257 = -2 ("Active Item:Row Number")
            n139 = Index Array(array=w251, index=w250) -> (element=w252:T23)
            n140 = Unbundle(w252) -> ("Operation"=w253:enum16{"Update", "Clear"}, "Color Box"=w254:u32)
            n141 = call <vilib>:"NT Read and Format Entries as Tree.vi"("Operation"=w253, "Name Pattern"=w258, "Tree Refnum"=w259) -> ()  [unwired: 7 in, 2 out]
            n142 = call <vilib>:"NT Read String.vi"("Name"="TestMode/TestName") -> ("String"=w248:string)  [unwired: 9 in, 1 out]
            n143 = case shown="\"\"" w248 {
              tunnel: "TestMode/TestProgress" ("Name") -> [w261 _]
              tunnel: "TestMode/TestProgressText" ("Name") -> [w260 _]
              frame Default {
                n144 = call <vilib>:"NT Read Number.vi"("Name"=w261) -> ("Numeric"=w262:dbl)  [unwired: 9 in, 1 out]
                n145 = call <vilib>:"NT Read String.vi"("Name"=w260) -> ("String"=w263:string)  [unwired: 9 in, 1 out]
                n146 = Bundle("Numeric"=w262, "String"=w263) -> (→"Progress":cluster{"Numeric":dbl, "String":string})  [unwired: 1 in]
              }
              frame "" {
                n147 = local write "Test Name"(u16 0) -> ()
                n148 = property on="Progress" class="Clust (strict)"("Visible"=FALSE) -> ()  [unwired: 2 in, 2 out]
              }
            }
            n149 = property on="Test Tree" class="Tree (strict)"("Active Item Row Number"=w257, "ActiveColNum"=w257, "CellBG"=w254, "Active Item Row Number"=-1 ("Active Item:Row Number"), "CellBG"=u32 5789784 ("Color Box")) -> ()  [unwired: 2 in, 2 out]
          }
          frame "Variables" {
            w269 = string[] ["CameraPublisher", "Usage", "DB"]  # Items to initially close
            n150 = First Call?() -> (First Call?: T/F=w270:bool)
            n151 = control-ref of="Tree"() -> (w271:refnum<vi>)
            n152 = Select(t=w269, s=w270, f=string[] []) -> (s? t:f=w267:string[])
            n153 = call <vilib>:"NT Read and Format Entries as Tree.vi"("Tags to  Close"=w267, "Tree Refnum"=w271) -> ()  [unwired: 8 in, 2 out]
          }
          frame "Commands" {
            w280 = u32 5789784 ("Color Box")
            w281 = T24 {"Row"=-1, "Column"=-2} ("Active Cell:Active Cell")
            w283 = T24 {"Row"=-2, "Column"=-2} ("Active Cell:Active Cell")
            n154 = Index Array(array=w279, index=w278) -> (element=w277:T23)
            n155 = Index Array(array=w284, index=w278) -> (element=w282:u32)
            n156 = local read "Command Selection"() -> (w275:i32)
            n157 = property on="Command Selection" class="MCListbox (strict)"("ActiveCell"=w283, "CellBG"=w282, "ActiveCell"=w281, "CellBG"=w280) -> ()  [unwired: 2 in, 2 out]
            n158 = property on="Command Params" class="Tbl (strict)"("Active Cell"=w283, "Cell BG Color"=w282, "Active Cell"=w281, "Cell BG Color"=w280) -> ()  [unwired: 2 in, 2 out]
            n159 = Unbundle(w277) -> ("Operation"=w276:enum16{"Update", "Clear"})  [unwired: 1 out]
            n160 = call <vilib>:"WPI_DashboardUpdate RPC Info.vi"("Operation"=w276) -> ("update"=w274:bool, "commands"=w273:string[][])  [unwired: 9 in]
            n161 = call <vilib>:"WPI_DashboardUpdate Command Params.vi"("Update"=w274, "NewVal"=w275, "Commands"=w273, "Param Tbl"=w272) -> ()  [unwired: 7 in, 1 out]
            n162 = property on="Command Selection" class="MCListbox (strict)"("ItemNames"=w273) -> ()  [unwired: 2 in, 2 out]
          }
        }
      }
      event "Test Tree": Value Change {
        # "Show appropriate\ncontrols"
        n163 = event-data() -> ("CtlRef"=w289:refnum<vi>, "NewVal"=w287:string)  [unwired: 1 in]
        n164 = call <vilib>:"WPI_UtilitiesGetTreeIOName.vi"("NewVal"=w287, "TreeControl in"=w289) -> ("I/O Name"=w290:string)  [unwired: 9 in]
        n165 = property on="Progress" class="Clust (strict)"("Visible"=FALSE) -> ()  [unwired: 2 in, 2 out]
        n166 = case shown="\"Camera\"" w290 {
          selector: w290 -> [_ w297 _ w319 w328 _]
          tunnel: w287 -> [_ _ w316 w318 _ w335]
          tunnel: cluster{string[]}[] [{["640x480", "320x240", "160x120"]}, {["Auto", "Fixed indoor", "Fixed outdoor 1", "Fixed outdoor 2", "Fixed fluorescent 1", "Fixed fluorescent 2", "Hold current"]}, {["Auto", "Flicker-free 50 Hz", "Flicker-free 60 Hz", "Hold current"]}, {["None", "Prioritize frame rate", "Prioritize image quality"]}, {["Monochrome", "Color"]}] -> [_ _ _ _ _ w334]
          frame Default {
            w292 = FALSE ("Visible")
            w291 = FALSE ("Visible")
            n167 = property on="Test Slider" class="Slide (strict)"("Visible"=w292) -> ()  [unwired: 2 in, 2 out]
            n168 = property on="On/Off" class="Bool (strict)"("Visible"=w292) -> ()  [unwired: 2 in, 2 out]
            n169 = property on="Rev/Fwd" class="Clust (strict)"("Visible"=w292) -> ()  [unwired: 2 in, 2 out]
            n170 = property on="Test Ring" class="Ring (strict)"("Visible"=w291) -> ()  [unwired: 2 in, 2 out]
            n171 = property on="Motor" class="Clust (strict)"("Visible"=w291) -> ()  [unwired: 2 in, 2 out]
          }
          frame "Analog Out", "Motor", "PWM" {
            w298 = FALSE ("Visible")
            n172 = case shown="\"Analog Out\"" w297 {
              tunnel: [1.0 ("Value") -1.0 ("Value") 0.0 ("Value")] -> w296
              tunnel: [255.0 ("Value") 1.0 ("Value") 5.0 ("Value")] -> w295
              tunnel: [128.0 ("Value") 0.0 ("Value") 0.0 ("Value")] -> w294
              tunnel: [64.0 ("Value") 0.5 ("Value") 1.0 ("Value")] -> w293
              frame "PWM" {
              }
              frame "Motor", Default {
              }
              frame "Analog Out" {
              }
            }
            n173 = property on="Motor" class="Clust (strict)"("Visible"=TRUE) -> ()  [unwired: 2 in, 2 out]
            n174 = property on="Test Slider" class="Slide (strict)"("Visible"=w298) -> ()  [unwired: 2 in, 2 out]
            n175 = property on="Test Ring" class="Ring (strict)"("Visible"=w298) -> ()  [unwired: 2 in, 2 out]
            n176 = property on="On/Off" class="Bool (strict)"("Visible"=w298) -> ()  [unwired: 2 in, 2 out]
            n177 = property on="Rev/Fwd" class="Clust (strict)"("Visible"=w298) -> ()  [unwired: 2 in, 2 out]
            n178 = property on="Value" class="Slide (strict)"("Value"=w294, "Scale.Minimum"=w296, "Scale.Maximum"=w295, "Scale.Increment"=w293) -> ()  [unwired: 2 in, 2 out]
          }
          frame "Servo" {
            w314 = FALSE ("Visible")
            n179 = call <vilib>:"NT Read Number.vi"("Name"=w316) -> ("Numeric"=w315:dbl)  [unwired: 9 in, 1 out]
            n180 = property on="Motor" class="Clust (strict)"("Visible"=w314) -> ()  [unwired: 2 in, 2 out]
            n181 = property on="Test Ring" class="Ring (strict)"("Visible"=w314) -> ()  [unwired: 2 in, 2 out]
            n182 = property on="On/Off" class="Bool (strict)"("Visible"=w314) -> ()  [unwired: 2 in, 2 out]
            n183 = property on="Rev/Fwd" class="Clust (strict)"("Visible"=w314) -> ()  [unwired: 2 in, 2 out]
            n184 = property on="Test Slider" class="Slide (strict)"("Visible"=TRUE, "Scale.Maximum"=170.0 ("Scale.Range:Maximum")) -> ()  [unwired: 2 in, 2 out]
            n185 = local write "Test Slider"(w315) -> ()
          }
          frame "Relay", "Solenoid" {
            w317 = FALSE ("Visible")
            n186 = property on="Motor" class="Clust (strict)"("Visible"=w317) -> ()  [unwired: 2 in, 2 out]
            n187 = property on="Test Slider" class="Slide (strict)"("Visible"=w317) -> ()  [unwired: 2 in, 2 out]
            n188 = property on="Test Ring" class="Ring (strict)"("Visible"=w317) -> ()  [unwired: 2 in, 2 out]
            n189 = Search and Replace String(input string=w318, search string="/Value  **", replace string="/Direction") -> (result string=w324:string)  [unwired: 5 in, 3 out]
            n190 = call <vilib>:"NT Read String.vi"("Name"=w324) -> ("String"=w322:string)  [unwired: 9 in, 1 out]
            n191 = Equal?(x="Both directions", y=w322) -> (x = y?=w320:bool)
            n192 = property on="Rev/Fwd" class="Clust (strict)"("Visible"=w320) -> ()  [unwired: 2 in, 2 out]
            n193 = Not(x=w320) -> (.not. x?=w321:bool)
            n194 = property on="On/Off" class="Bool (strict)"("Visible"=w321, "Caption.Text"=w319) -> ()  [unwired: 2 in, 2 out]
          }
          frame "Compressor", "Digital Out" {
            w327 = FALSE ("Visible")
            # "Get direction and finish"
            n195 = property on="Rev/Fwd" class="Clust (strict)"("Visible"=FALSE) -> ()  [unwired: 2 in, 2 out]
            n196 = property on="Test Ring" class="Ring (strict)"("Visible"=w327) -> ()  [unwired: 2 in, 2 out]
            n197 = property on="Motor" class="Clust (strict)"("Visible"=w327) -> ()  [unwired: 2 in, 2 out]
            n198 = property on="Test Slider" class="Slide (strict)"("Visible"=w327) -> ()  [unwired: 2 in, 2 out]
            n199 = property on="On/Off" class="Bool (strict)"("Visible"=TRUE, "Caption.Text"=w328) -> ()  [unwired: 2 in, 2 out]
          }
          frame "Camera" {
            n200 = call <vilib>:"Get Last Path Segment.vi"("String in"=w335) -> ("String out"=w336:string)  [unwired: 10 in]
            n201 = property on="On/Off" class="Bool (strict)"("Visible"=FALSE) -> ()  [unwired: 2 in, 2 out]
            n202 = property on="Rev/Fwd" class="Clust (strict)"("Visible"=FALSE) -> ()  [unwired: 2 in, 2 out]
            n203 = case shown="\"White Balance  **\"" w336 {
              tunnel: w335 -> [w342 w351 w360 w369 w378 _ w384]
              tunnel: w334 -> [w340 w348 w357 w366 w375 _ _]
              frame "Size  **" {
                n204 = Index Array(array=w340) -> (element=w339:cluster{string[]})  [unwired: 1 in]
                n205 = call <vilib>:"NT Read String.vi"("Name"=w342) -> ("String"=w341:string)  [unwired: 9 in, 1 out]
                n206 = property on="Test Slider" class="Slide (strict)"("Visible"=FALSE) -> ()  [unwired: 2 in, 2 out]
                n207 = property on="Test Ring" class="Ring (strict)"("Visible"=TRUE) -> ()  [unwired: 2 in, 2 out]
                n208 = Unbundle(w339) -> (w337:string[])
                n209 = Match First String(2:w337, 3:w341) -> (0:w338:i32)  [unwired: 1 out]
                n210 = property on="Test Ring" class="Ring (strict)"("Value"=w338, "Strings []"=w337) -> ()  [unwired: 2 in, 2 out]
              }
              frame "White Balance  **" {
                n211 = call <vilib>:"NT Read String.vi"("Name"=w351) -> ("String"=w350:string)  [unwired: 9 in, 1 out]
                n212 = Index Array(array=w348, index=1) -> (element=w349:cluster{string[]})
                n213 = property on="Test Slider" class="Slide (strict)"("Visible"=FALSE) -> ()  [unwired: 2 in, 2 out]
                n214 = property on="Test Ring" class="Ring (strict)"("Visible"=TRUE) -> ()  [unwired: 2 in, 2 out]
                n215 = Unbundle(w349) -> (w346:string[])
                n216 = Match First String(2:w346, 3:w350) -> (0:w345:i32)  [unwired: 1 out]
                n217 = property on="Test Ring" class="Ring (strict)"("Value"=w345, "Strings []"=w346) -> ()  [unwired: 2 in, 2 out]
              }
              frame "Exposure  **" {
                n218 = call <vilib>:"NT Read String.vi"("Name"=w360) -> ("String"=w359:string)  [unwired: 9 in, 1 out]
                n219 = Index Array(array=w357, index=2) -> (element=w358:cluster{string[]})
                n220 = property on="Test Slider" class="Slide (strict)"("Visible"=FALSE) -> ()  [unwired: 2 in, 2 out]
                n221 = property on="Test Ring" class="Ring (strict)"("Visible"=TRUE) -> ()  [unwired: 2 in, 2 out]
                n222 = Unbundle(w358) -> (w354:string[])
                n223 = Match First String(2:w354, 3:w359) -> (0:w355:i32)  [unwired: 1 out]
                n224 = property on="Test Ring" class="Ring (strict)"("Value"=w355, "Strings []"=w354) -> ()  [unwired: 2 in, 2 out]
              }
              frame "Exposure Priority  **" {
                n225 = call <vilib>:"NT Read String.vi"("Name"=w369) -> ("String"=w368:string)  [unwired: 9 in, 1 out]
                n226 = Index Array(array=w366, index=3) -> (element=w367:cluster{string[]})
                n227 = property on="Test Slider" class="Slide (strict)"("Visible"=FALSE) -> ()  [unwired: 2 in, 2 out]
                n228 = property on="Test Ring" class="Ring (strict)"("Visible"=TRUE) -> ()  [unwired: 2 in, 2 out]
                n229 = Unbundle(w367) -> (w363:string[])
                n230 = Match First String(2:w363, 3:w368) -> (0:w364:i32)  [unwired: 1 out]
                n231 = property on="Test Ring" class="Ring (strict)"("Value"=w364, "Strings []"=w363) -> ()  [unwired: 2 in, 2 out]
              }
              frame "Color Enable  **" {
                n232 = call <vilib>:"NT Read String.vi"("Name"=w378) -> ("String"=w377:string)  [unwired: 9 in, 1 out]
                n233 = Index Array(array=w375, index=4) -> (element=w376:cluster{string[]})
                n234 = property on="Test Slider" class="Slide (strict)"("Visible"=FALSE) -> ()  [unwired: 2 in, 2 out]
                n235 = property on="Test Ring" class="Ring (strict)"("Visible"=TRUE) -> ()  [unwired: 2 in, 2 out]
                n236 = Unbundle(w376) -> (w372:string[])
                n237 = Match First String(2:w372, 3:w377) -> (0:w373:i32)  [unwired: 1 out]
                n238 = property on="Test Ring" class="Ring (strict)"("Value"=w373, "Strings []"=w372) -> ()  [unwired: 2 in, 2 out]
              }
              frame Default {
                n239 = property on="Test Slider" class="Slide (strict)"("Visible"=FALSE) -> ()  [unwired: 2 in, 2 out]
                n240 = property on="Test Ring" class="Ring (strict)"("Visible"=FALSE) -> ()  [unwired: 2 in, 2 out]
              }
              frame "Brightness  **", "Color Level  **", "Compression  **", "FPS  **", "Sharpness  **" {
                n241 = call <vilib>:"NT Read Number.vi"("Name"=w384) -> ("Numeric"=w383:dbl)  [unwired: 9 in, 1 out]
                n242 = property on="Test Ring" class="Ring (strict)"("Visible"=FALSE) -> ()  [unwired: 2 in, 2 out]
                n243 = property on="Test Slider" class="Slide (strict)"("Visible"=TRUE, "Scale.Maximum"=100.0 ("Scale.Range:Maximum")) -> ()  [unwired: 2 in, 2 out]
                n244 = local write "Test Slider"(w383) -> ()
              }
            }
            n245 = property on="Motor" class="Clust (strict)"("Visible"=FALSE) -> ()  [unwired: 2 in, 2 out]
          }
        }
      }
      event "Test Name": Mouse Enter {
        # "Populate the ring with the list of tests"
        n246 = event-data() -> ()  [unwired: 1 in, 1 out]
        n247 = call <vilib>:"NT Read String Array.vi"("Name"="TestMode/TestList") -> ("String Array"=w392:string[])  [unwired: 9 in, 1 out]
        n248 = Build Array (concatenate)("Select the test to run...", w392) -> (w391:string[])
        n249 = property on="Test Name" class="Ring (strict)"("Strings []"=w391) -> ()  [unwired: 2 in, 2 out]
      }
      event "Test Name": Value Change {
        w394 = FALSE ("Visible")
        # "Tell the robot the test name to run"
        n250 = event-data() -> ("NewVal"=w398:u16)  [unwired: 1 in]
        n251 = property on="Test Name" class="Ring (strict)"() -> ("Strings []"=w399:string[])  [unwired: 2 in, 2 out]
        n252 = property on="Test Ring" class="Ring (strict)"("Visible"=w394) -> ()  [unwired: 2 in, 2 out]
        n253 = property on="Motor" class="Clust (strict)"("Visible"=w394) -> ()  [unwired: 2 in, 2 out]
        n254 = property on="Test Slider" class="Slide (strict)"("Visible"=w394) -> ()  [unwired: 2 in, 2 out]
        n255 = property on="On/Off" class="Bool (strict)"("Visible"=w394) -> ()  [unwired: 2 in, 2 out]
        n256 = property on="Rev/Fwd" class="Clust (strict)"("Visible"=w394) -> ()  [unwired: 2 in, 2 out]
        n257 = property on="Progress" class="Clust (strict)"("Visible"=TRUE) -> ()  [unwired: 2 in, 2 out]
        n258 = local write "Progress"(T6 {"Test Progress"=0, "Test Progress Text"=""} ("Progress")) -> ()
        n259 = Index Array(array=w399, index=w398) -> (element=w397:string)
        n260 = call <vilib>:"NT Write String.vi"("String"=w397, "Name"="TestMode/TestName") -> ()  [unwired: 9 in, 1 out]
      }
      event "Select Auto": Mouse Enter {
        # "Populate the combo box with the list of autonomous options"
        n261 = event-data() -> ()  [unwired: 1 in, 1 out]
        n262 = call <vilib>:"NT Read String Array.vi"("Name"="Auto List") -> ("String Array"=w401:string[])  [unwired: 9 in, 1 out]
        n263 = property on="Select Auto" class="CmbBox"("Strings[]"=w401) -> ()  [unwired: 2 in, 2 out]
      }
      event "Select Auto": Value Change {
        # "User modified the Auto Selection. Write to NT variable so robot knows."
        n264 = event-data() -> ("NewVal"=w404:string)  [unwired: 1 in]
        n265 = call <vilib>:"NT Write String.vi"("String"=w404, "Name"="Auto Selector") -> ()  [unwired: 9 in, 1 out]
      }
      event "Command Selection": Value Change {
        # "Get the params and show in table"
        n266 = event-data() -> ("NewVal"=w410:i32)  [unwired: 1 in]
        n267 = property on="Command Selection" class="MCListbox (strict)"() -> ("ItemNames"=w408:string[][])  [unwired: 2 in, 2 out]
        n268 = call <vilib>:"WPI_DashboardUpdate Command Params.vi"("NewVal"=w410, "Commands"=w408, "Param Tbl"=w409) -> ()  [unwired: 8 in, 1 out]
      }
      event "Execute Command": Value Change {
        # "Started one, Unique ID holds\nresponse"
        n269 = event-data() -> ()  [unwired: 1 in, 1 out]
        n270 = property on="Command Selection" class="MCListbox (strict)"() -> ("ItemNames"=w421:string[][])  [unwired: 2 in, 2 out]
        n271 = Index Array(array=w421, index (row)="Command Selection", index (col)=0) -> (element=w419:string)
        n272 = call <vilib>:"Invoke Commands.vi"("Command Params"="Command Params", "Function Name"=w419) -> ("Params"=w415:u8, "Started"=w414:bool)  [unwired: 7 in, 1 out]
        n273 = Array Subset(array="Command Params", length (row)=w415) -> (w416:string[][])  [unwired: 3 in]
        n274 = Select(t="Executing" ("Cmd Status"), s=w414, f="" ("Cmd Status")) -> (s? t:f=→"Cmd Status":string)
      }
      event "Command Selection": Double Click {
        n275 = event-data() -> ("Row"=w429:i32)  [unwired: 1 in]
        n276 = property on="Command Selection" class="MCListbox (strict)"() -> ("ItemNames"=w432:string[][])  [unwired: 2 in, 2 out]
        n277 = local read "Command Params"() -> (w428:string[][])
        n278 = Index Array(array=w432, index (row)=w429, index (col)=0) -> (element=w430:string)
        n279 = call <vilib>:"Invoke Commands.vi"("Command Params"=w428, "Function Name"=w430) -> ("Params"=w427:u8, "Started"=w422:bool)  [unwired: 7 in, 1 out]
        n280 = Array Subset(array=w428, length (row)=w427) -> (w426:string[][])  [unwired: 3 in]
        n281 = Select(t="Executing" ("Cmd Status"), s=w422, f="" ("Cmd Status")) -> (s? t:f=w423:string)
        n282 = local write "Cmd Status"(w423) -> ()
      }
      event "CheckList": Double Click {
        # "Shift clears all"
        # "Update symbols on the listbox"
        n283 = event-data() -> ("PlatMods.Shift"=w434:bool, "Row"=w436:i32)  [unwired: 1 in]
        n284 = case shown="True" w434 {
          tunnel: w436 -> [w440 _]
          tunnel: 1 -> [w439 _]
          frame False {
            n285 = property on="CheckList" class="LstBox (strict)"() -> ("Item Symbols"=w438:i32[])  [unwired: 2 in, 2 out]
            n286 = Replace Array Subset(array=w438, new element=w439, index=w440) -> (w437:i32[])
            n287 = property on="CheckList" class="LstBox (strict)"("Item Symbols"=w437) -> ()  [unwired: 2 in, 2 out]
          }
          frame True {
            w441 = 0 ("Top Row")
            n288 = property on="CheckList" class="LstBox (strict)"() -> ("Number of Rows"=w443:u32)  [unwired: 2 in, 2 out]
            n289 = Initialize Array(0, w443) -> (w442:i32[])
            n290 = property on="CheckList" class="LstBox (strict)"("Top Row"=w441, "Value"=w441, "Item Symbols"=w442) -> ()  [unwired: 2 in, 2 out]
          }
        }
      }
      event "CheckList": Key Down {
        # "Update symbols on the listbox\nLeft and right keys check and uncheck"
        n291 = event-data() -> ("VKey"=w447:T21)  [unwired: 1 in]
        n292 = case shown="\"Left\", \"Right\"" w447 {
          selector: w447 -> [w452 _]
          tunnel: eventvkey."Left" ("VKey") -> [w450 _]
          frame "Left", "Right" {
            n293 = Equal?(x=w450, y=w452) -> (x = y?=w451:bool)
            n294 = Select(t=0, s=w451, f=1) -> (s? t:f=w453:i32)
            n295 = property on="CheckList" class="LstBox (strict)"() -> ("Item Symbols"=w456:i32[])  [unwired: 2 in, 2 out]
            n296 = Replace Array Subset(array=w456, new element=w453, index="CheckList") -> (w455:i32[])
            n297 = property on="CheckList" class="LstBox (strict)"("Item Symbols"=w455) -> ()  [unwired: 2 in, 2 out]
          }
          frame Default {
          }
        }
      }
      event "Motor.Enable": Value Change {
        # "When the test mode otor enable helper is set, update that\ntree row item's value"
        n298 = event-data() -> ("NewVal"=w462:bool)  [unwired: 1 in]
        n299 = Unbundle("Motor") -> ("Value"=w461:dbl)  [unwired: 1 out]
        n300 = Select(t=w461, s=w462, f=0.0) -> (s? t:f=w459:dbl)
        n301 = call <vilib>:"NT Write Number.vi"("Numeric"=w459, "Name"=w458) -> ()  [unwired: 9 in, 1 out]
      }
      event "Test Slider": Value Change {
        # "When the test mode slider helper is set, update that\ntree row item's value"
        n302 = event-data() -> ("NewVal"=w465:dbl)  [unwired: 1 in]
        n303 = call <vilib>:"NT Write Number.vi"("Numeric"=w465, "Name"=w466) -> ()  [unwired: 9 in, 1 out]
      }
      event "On/Off": Value Change {
        # "When the test mode on/off helper value is set, update that\ntree row item's value"
        n304 = event-data() -> ("NewVal"=w470:bool)  [unwired: 1 in]
        n305 = Boolean To (0,1)(Boolean=w470) -> (0, 1=w469:i16)
        n306 = call <vilib>:"NT Write Number.vi"("Numeric"=w469, "Name"=w468) -> ()  [unwired: 9 in, 1 out]
      }
      event "Rev/Fwd": Value Change {
        # "When the test mode helper value for relays is set, update that\ntree row item's value"
        n307 = event-data() -> ("NewVal.Forward"=w478:bool, "NewVal.Reverse"=w477:bool)  [unwired: 1 in]
        n308 = Boolean To (0,1)(Boolean=w478) -> (0, 1=w474:i16)
        n309 = Boolean To (0,1)(Boolean=w477) -> (0, 1=w476:i16)
        n310 = Negate(x=w476) -> (-x=w475:i16)
        n311 = Add(x=w474, y=w475) -> (x+y=w473:i16)
        n312 = call <vilib>:"NT Write Number.vi"("Numeric"=w473, "Name"=w472) -> ()  [unwired: 9 in, 1 out]
      }
      event "Test Ring": Value Change {
        # "When a test mode helper value is selected from the ring,\nset the tree item's variable to the string value"
        n313 = event-data() -> ("NewVal"=w482:u16)  [unwired: 1 in]
        n314 = property on="Test Ring" class="Ring (strict)"() -> ("Strings []"=w483:string[])  [unwired: 2 in, 2 out]
        n315 = Index Array(array=w483, index=w482) -> (element=w481:string)
        n316 = call <vilib>:"NT Write String.vi"("String"=w481, "Name"=w480) -> ()  [unwired: 9 in, 1 out]
      }
      event "Rec Mode": Value Change {
        # "Update globals for recording mode and path to read log from.\nClear when logging and let NetworkTables set path for vision to\nuse."
        n317 = event-data() -> ("NewVal"=w494:enum32{"Stop", "Record", "Playback"})  [unwired: 1 in]
        n318 = global write "WPI_DashboardLogging Global.vi" "Recording"(w494) -> ()
        n319 = global write "WPI_DashboardLogging Global.vi" "Logging Filename"(path "") -> ()
        n320 = case shown="\"Playback\"" w494 {
          tunnel: w493 -> [_ w496 w505]
          tunnel: [_ _ w504] -> w491
          tunnel: [_ _ w503] -> _
          tunnel: w489 -> [_ _ w501]
          tunnel: cluster{i32, i32} {-250, 170} -> [_ _ w500]
          tunnel: [_ _ T22 {"Image Size"=TRUE, "Image Type"=TRUE, "Pixel Value"=TRUE, "ROI Information"=TRUE, "Zoom Factor"=FALSE} ("Image Information Shown:All Elements")] -> w484
          tunnel: [_ _ TRUE ("Zoom Factor")] -> w485
          tunnel: w487 -> [_ _ w497]
          frame Default {
          }
          frame "Stop", "Record" {
            # "Place Window too"
            n321 = invoke class="VI" method="FP.Close"(reference=w496) -> (reference out=w495:refnum<vi>)  [unwired: 2 in, 2 out]
            n322 = invoke class="VI" method="Abort VI"(reference=w495) -> ()  [unwired: 2 in, 3 out]
          }
          frame "Playback" {
            n323 = call "Open Playback Panel.vi"("Offset"=w500, "DB VI Ref"=w501, "Playback in"=w505) -> ("Playback out"=w502:refnum<vi>)  [unwired: 8 in]
            n324 = register-events(w502, w497) -> (reference out=w504:refnum<event-registration>, error out=w503:errorcluster)  [unwired: 2 in]
          }
        }
        n325 = call <vilib>:"WPI_DashboardNT Log FieldName Cache.vi"("Operation"=enum16{"Lookup/Add", "Index", "Clear"}."Clear") -> ()  [unwired: 8 in, 3 out]
        n326 = property on="Camera Image" class="ImageControl"("Image Information Shown"=w484, "Image Information Visible"=w485) -> ()  [unwired: 2 in, 2 out]
        n327 = property on="Camera Image Right" class="ImageControl"("Image Information Shown"=w484, "Image Information Visible"=w485) -> ()  [unwired: 2 in, 2 out]
      }
      event Panel Close {
        w507 = enum32{"Stop", "Record", "Playback"}."Stop" ("Rec Mode")
        # "Playback window has been closed, abort"
        n328 = event-data() -> ()  [unwired: 1 in, 4 out]
        n329 = local write "Rec Mode"(w507) -> ()
        n330 = global write "WPI_DashboardLogging Global.vi" "Recording"(w507) -> ()
      }
      event Panel Close {
        # "Abort playback window and ourself"
        n331 = event-data() -> ()  [unwired: 1 in, 4 out]
        n332 = invoke class="VI" method="FP.Close"(reference=w511) -> (reference out=w510:refnum<vi>)  [unwired: 2 in, 2 out]
        n333 = invoke class="VI" method="Abort VI"(reference=w510) -> (error out=w509:errorcluster)  [unwired: 2 in, 2 out]
        n334 = invoke class="VI" method="Abort VI"(error in=w509) -> ()  [unwired: 2 in, 3 out]
      }
      event User Event {
        n335 = event-data() -> ("IDs"=w518:cluster{"RPC field ID":u16, "Unique ID":u16}, "String"=w517:string)  [unwired: 1 in]
        n336 = Bundle("IDs"=w518, "String"=w517) -> (w516:T9)  [unwired: 1 in]
        n337 = local write "Cmd Status"("" ("Cmd Status")) -> ()
        n338 = call <vilib>:"Retrieve RPC Response.vi"("RPC Response"=w516) -> ("Output"=w514:string[][])  [unwired: 10 in]
        n339 = Build Array (concatenate)(w512, w514) -> (w513:string[][])
        n340 = local write "Command Params"(w513) -> ()
      }
      event "Tree": Double Click {
        n341 = event-data() -> ("PlatMods"=w524:T25, "Tag"=w521:string)  [unwired: 1 in]
        n342 = Unbundle(w524) -> ("Shift"=w523:bool)  [unwired: 4 out]
        n343 = Not(x=w523) -> (.not. x?=w522:bool)
        n344 = String Subset(string=w521, length (rest)=1 ("length (rest)")) -> (substring=w520:string)  [unwired: 1 in]
        n345 = case shown="\"/\"" w520 {
          tunnel: w521 -> [_ w527]
          tunnel: w522 -> [_ w526]
          frame Default {
          }
          frame "/" {
            n346 = call <vilib>:"NT Update Persistence.vi"("Persistence"=w526, "Name"=w527) -> ()  [unwired: 9 in, 1 out]
          }
        }
      }
    }
  }
